vi "DrawRectAndShowRectName.vi"(1 "String":string, 2 "Img in":T1, 3 "ROI":T2 {"Contours"."Type" items=["No Selection", "Point", "Line", "Rectangle", "Oval", "Polygon", "Free", "Annulus", "Unused2", "Unused3", "Broken Line", "Free Hand Line", "Rotated Rectangle"]}) -> ()   [LabVIEW 2014]
uses:
  <vilib>/vision/Image Controls.llb/IMAQ Image.ctl
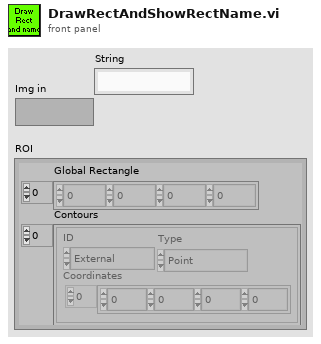
[diagram p1: front panel]
types:
  T1 = typedef "IMAQ Image.ctl" = refnum<image>
  T2 = cluster{"Global Rectangle":i32[], "Contours":cluster{"ID":enum32{"External", "Internal"}, "Type":u32, "Coordinates":i32[]}[]}
  T3 = cluster{"Desired Font (Application)":enum16{"User-specified Font", "Application Font", "System Font", "Dialog Font"}, "[User-specified Font]":cluster{"Font Name":string, "Size":i16, "Strikeout?":bool, "Italic?":bool, "Underline?":bool, "Outline?":bool, "Shadow?":bool, "Bold?":bool, "Rotation Angle":dbl}, "Horizontal Alignment":i16, "Vertical Alignment":i16}
  T4 = cluster{"ID":enum32{"External", "Internal"}, "Type":u32, "Coordinates":i32[]}[]
  T5 = cluster{"ID":enum32{"External", "Internal"}, "Type":u32, "Coordinates":i32[]}
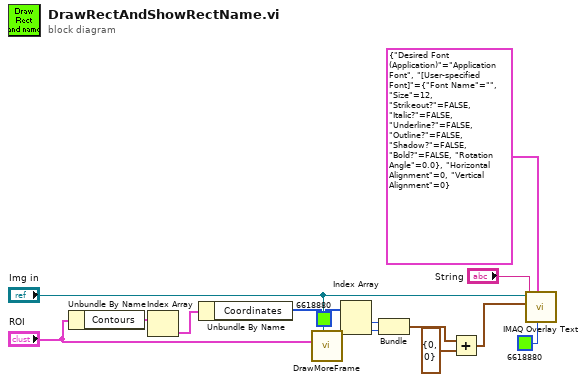
[diagram p0: block diagram]
diagram:
  n1 = Unbundle By Name("ROI") -> ("Contours"=w3:T4)
  n2 = Index Array(array=w3) -> (element=w2:T5)  [unwired: 1 in]
  n3 = Unbundle By Name(w2) -> ("Coordinates"=w1:i32[])
  n4 = call "DrawMoreFrame.vi"("ROI"="ROI", "Color"=u32 6618880, "Image Out 2"="Img in") -> ()  [unwired: 4 in, 1 out]
  n5 = Index Array(array=w1) -> (element #1=w10:i32, element #2=w11:i32)  [unwired: 2 in]
  n6 = Bundle(w10, w11) -> (w6:cluster{i32, i32})  [unwired: 1 in]
  n7 = Add(x=w6, y=cluster{i32, i32} {0, 0}) -> (x+y=w4:cluster{i32, i32})
  n8 = call "IMAQ Overlay Text"("Text Color (black)"=u32 6618880, "Font, Size & Style"=T3 {"Desired Font (Application)"=enum."Application Font", "[User-specified Font]"={"Font Name"="", "Size"=12, "Strikeout?"=FALSE, "Italic?"=FALSE, "Underline?"=FALSE, "Outline?"=FALSE, "Shadow?"=FALSE, "Bold?"=FALSE, "Rotation Angle"=0.0}, "Horizontal Alignment"=0, "Vertical Alignment"=0}, "String"="String", "Origin"=w4, "Image"="Img in") -> ()  [unwired: 5 in, 2 out]
